vi "demo - Simple Serial.vi"() -> ()   [LabVIEW 2024]
doc: "#vi_description \nSends a simple serial request and receives a response as as string of byte characters.\nModified NI Example.\nThetic Engineering Ltd."
uses:
  <vilib>/Instr/_visa.llb/VISA Configure Serial Port (Instr).vi
  Program Files (x86)/National Instruments/LabVIEW 2024/examples/Instrument IO/Serial/support/typedef - Serial Settings.ctl
panel:
  in  "Serial Settings":T1={"baud rate"=9600, "data bits"=8, "parity"=enum."None", "stop bits"=10, "flow control"=0} {"flow control" items=["None"=0, "XON/XOFF"=1, "RTS/CTS"=2, "DTR/DSR"=4]; "stop bits" items=["1.0"=10, "1.5"=15, "2.0"=20]; "data bits" min=5 max=8 step=1; "baud rate" items=["75"=75, "110"=110, "134"=134, "150"=150, "300"=300, "600"=600, "1200"=1200, "1800"=1800, "2400"=2400, "4800"=4800, "7200"=7200, "9600"=9600, "14400"=14400, "19200"=19200, "28800"=28800, "38400"=38400, "56000"=56000, "57600"=57600, "115200"=115200, "128000"=128000, "230400"=230400]}
  out "bytes read":u32
  in  "delay before read (ms)":u32=500
  out "Response":string
  in  "VISA resource name":refnum<visa-resource-name>="COM3"
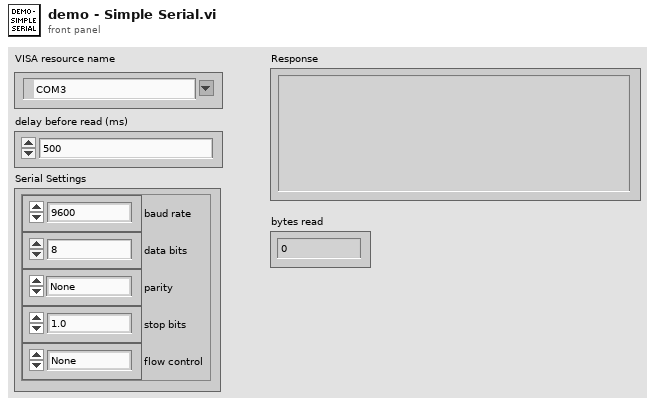
[diagram p1: front panel]
types:
  T1 = typedef "typedef - Serial Settings.ctl" = cluster{"baud rate":u32, "data bits":u16, "parity":enum16{"None", "Odd", "Even", "Mark", "Space"}, "stop bits":u16, "flow control":u16}
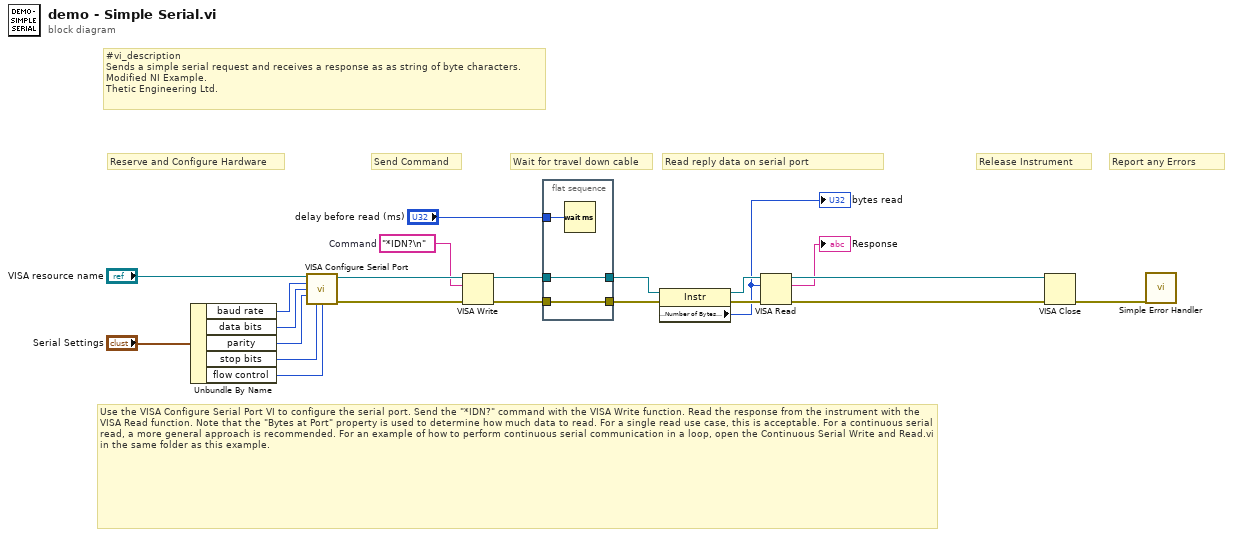
[diagram p0: block diagram]
diagram:
  w11 = "*IDN?\n"  # Command
  # "Report any Errors"
  # "Release Instrument"
  # "Read reply data on serial port"
  # "Wait for travel down cable"
  # "Send Command"
  # "Reserve and Configure Hardware"
  # "#vi_description \nSends a simple serial request and receives a response as as string of byte characters.\nModified NI Example.\nThetic Engineering Ltd."
  # "Use the VISA Configure Serial Port VI to configure the serial port. Send the \"*IDN?\" command with the VISA Write function. Read the response from the instrument with the VISA Read function. Note that the \"Bytes at Port\" property is used to determine how much data to read. For a single read use case, this is acceptable. For a continuous serial read, a more general approach is recommended. For an example of how to perform continuous serial communication in a loop, open the Continuous Serial Write and Read.vi in the same folder as this example."
  n1 = Unbundle By Name("Serial Settings") -> ("baud rate"=w5:u32, "data bits"=w4:u16, "parity"=w3:enum16{"None", "Odd", "Even", "Mark", "Space"}, "stop bits"=w2:u16, "flow control"=w1:u16)
  n2 = call-poly "VISA Configure Serial Port"("VISA resource name"="VISA resource name", "baud rate (9600)"=w5, "data bits (8)"=w4, "parity (0:none)"=w3, "stop bits (10: 1 bit)"=w2, "flow control (0:none)"=w1) -> ("VISA resource name out"=w20:refnum<visa-resource-name>, "error out"=w21:errorcluster)  [unwired: 3 in, 5 out]
  n3 = VISA Write(VISA resource name=w20, write buffer=w11, error in (no error)=w21) -> (VISA resource name out=w14:refnum<visa-resource-name>, error out=w16:errorcluster)  [unwired: 1 out]
  n4 = flat-sequence {
    tunnel: w16 -> [w24]
    tunnel: [w24] -> w15
    tunnel: w14 -> [w23]
    tunnel: [w23] -> w13
    tunnel: "delay before read (ms)" -> [w25]
    frame #0 {
      n5 = Wait (ms)(milliseconds to wait=w25) -> ()  [unwired: 1 out]
    }
  }
  n6 = property on="Property Node" class="Instr"(reference=w13, error in=w15) -> (reference out=w10:refnum<visa-resource-name>, error out=w9:errorcluster, "Serial Settings:Number of Bytes at Serial Port"=w7:u32)
  "bytes read" <- w7
  n7 = VISA Read(VISA resource name=w10, byte count=w7, error in (no error)=w9) -> (VISA resource name out=w18:refnum<visa-resource-name>, read buffer=→"Response":string, error out=w19:errorcluster)  [unwired: 1 out]
  n8 = VISA Close(VISA resource name=w18, error in (no error)=w19) -> (error out=w17:errorcluster)
  n9 = call <vilib>:"Simple Error Handler.vi"("error in (no error)"=w17) -> ()  [unwired: 1 in, 8 out]
